vi "KEVIN CREATE EMAIL.vi"(9 "DATA IN":T2, 10 "BYU ID # IN":string, 11 "connection reference in":T3) -> (2 "MESSAGE OUT":string, 3 "connection reference out":T3)   [LabVIEW 2019]
uses:
  <vilib>/addons/database/Connection.llb/Conn ObjectReference.ctl
  Controls/Table Data Types/Inventory Data Type.ctl
  Controls/Table Data Types/User Data Type.ctl
  <vilib>/addons/database/_DB Variant To Data/Database Variant To Data.xnode
  <vilib>/addons/database/NI_Database_API.lvlib
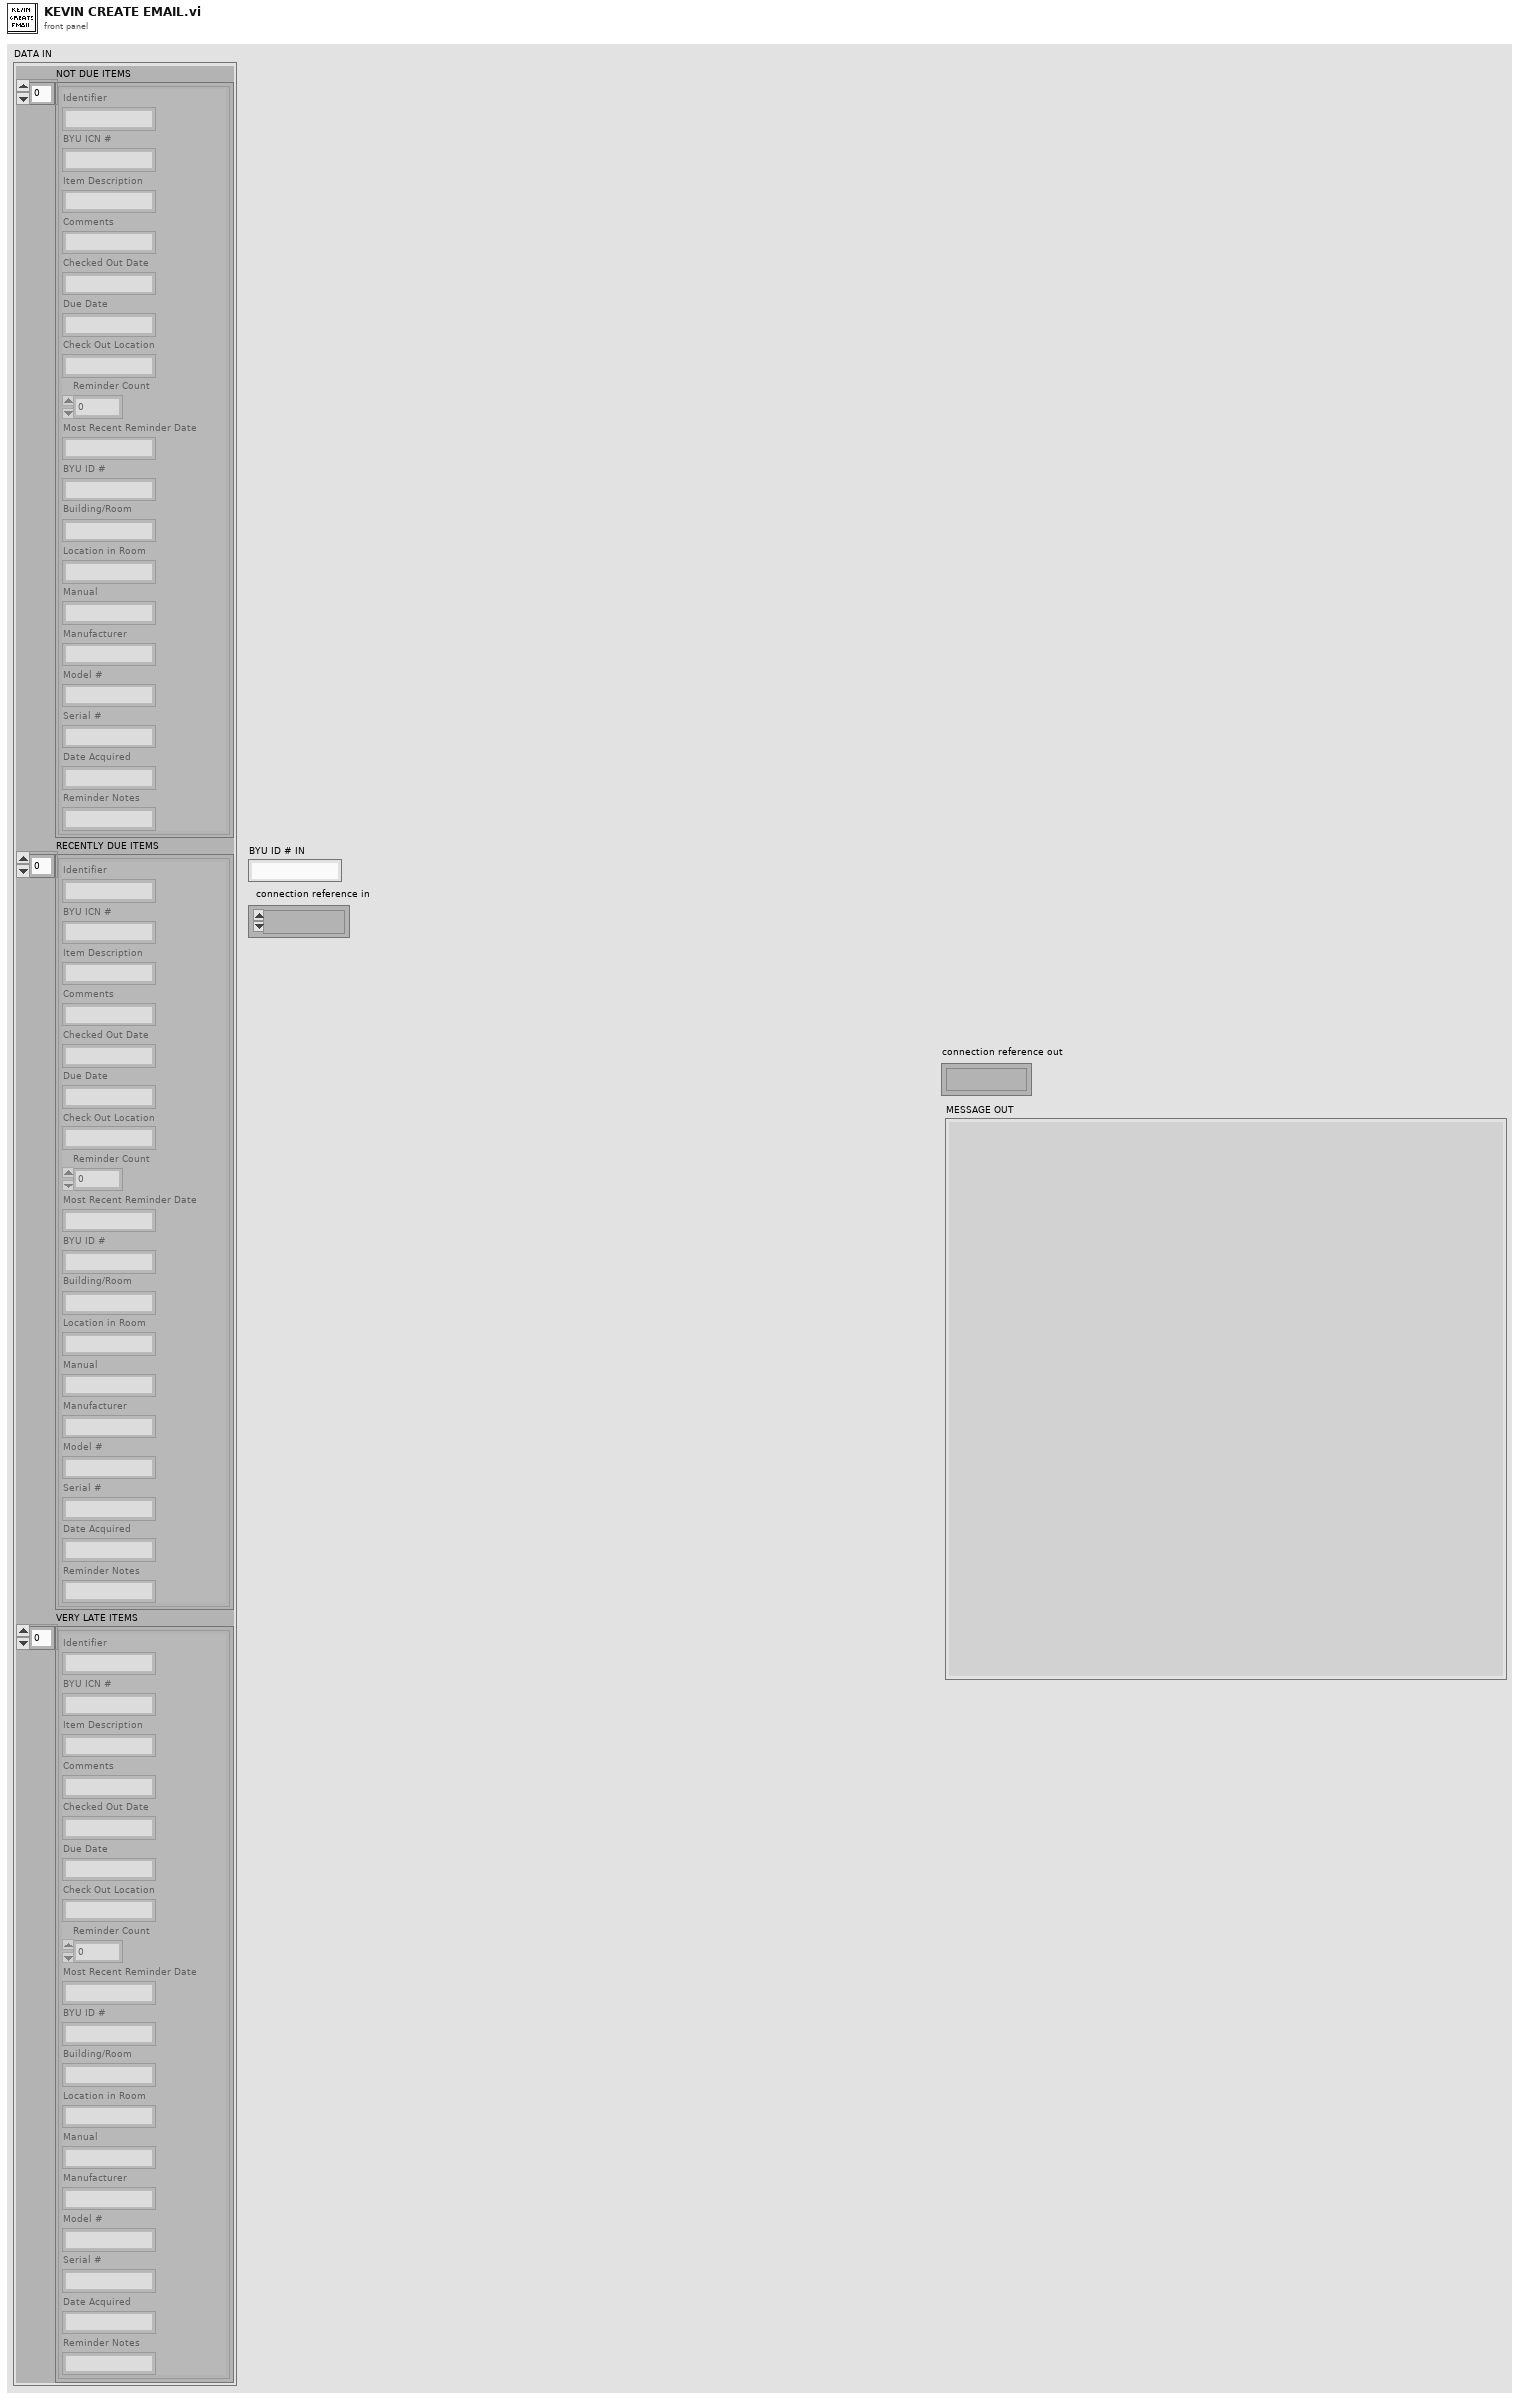
[diagram p1: front panel]
types:
  T1 = typedef "Inventory Data Type.ctl" = cluster{"Identifier":string, "BYU ICN #":string, "Item Description":string, "Comments":string, "Checked Out Date":string, "Due Date":string, "Check Out Location":string, "Reminder Count":i32, "Most Recent Reminder Date":string, "BYU ID #":string, "Building/Room":string, "Location in Room":string, "Manual":string, "Manufacturer":string, "Model #":string, "Serial #":string, "Date Acquired":string, "Reminder Notes":string}
  T2 = cluster{"NOT DUE ITEMS":T1[], "RECENTLY DUE ITEMS":T1[], "VERY LATE ITEMS":T1[]}
  T3 = typedef "NI_Database_API.lvlib/Conn ObjectReference.ctl" = refnum<k1>
  T4 = typedef "User Data Type.ctl" = cluster{"BYU ID #":string, "First Name":string, "Last Name":string, "Phone Number":string, "Email":string, "Department":string, "Graduation Status":string, "Anticipated Graduation Year":string, "Credit Score":dbl, "Date Added":string, "Graduation Clearance Date":string, "Picture File Name":string, "User Comments":string}
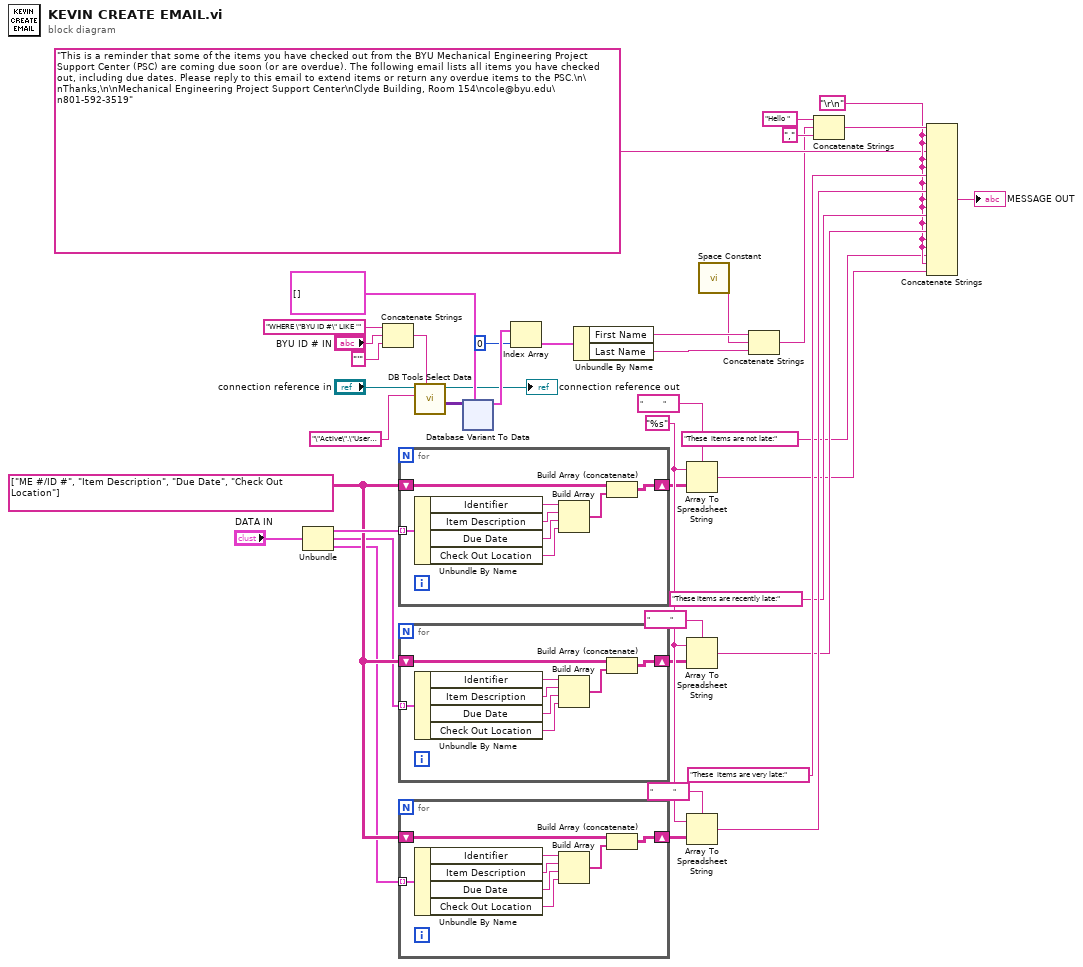
[diagram p0: block diagram]
diagram:
  w17 = "%s" ("table")
  w19 = "\r\n"
  w25 = string[][] [["ME #/ID #", "Item Description", "Due Date", "Check Out Location"]]
  n1 = Unbundle("DATA IN") -> ("NOT DUE ITEMS"=w26:T1[], "RECENTLY DUE ITEMS"=w3:T1[], "VERY LATE ITEMS"=w4:T1[])
  n2 = Concatenate Strings("WHERE \"BYU ID #\" LIKE '" ("table"), "BYU ID # IN", "'" ("table")) -> (w35:string)
  n3 = for {
    tunnel: w26 -> [w48] mode=indexing
    shift-right: [w41] -> w16
    shift-left: w25 -> [w43]
    n4 = Unbundle By Name(w48) -> ("Identifier"=w47:string, "Item Description"=w46:string, "Due Date"=w45:string, "Check Out Location"=w44:string)
    n5 = Build Array(w47, w46, w45, w44) -> (w42:string[])
    n6 = Build Array (concatenate)(w43, w42) -> (w41:string[][])
  }
  n7 = for {
    tunnel: w3 -> [w56] mode=indexing
    shift-right: [w49] -> w15
    shift-left: w25 -> [w51]
    n8 = Unbundle By Name(w56) -> ("Identifier"=w55:string, "Item Description"=w54:string, "Due Date"=w53:string, "Check Out Location"=w52:string)
    n9 = Build Array(w55, w54, w53, w52) -> (w50:string[])
    n10 = Build Array (concatenate)(w51, w50) -> (w49:string[][])
  }
  n11 = for {
    tunnel: w4 -> [w64] mode=indexing
    shift-right: [w57] -> w14
    shift-left: w25 -> [w59]
    n12 = Unbundle By Name(w64) -> ("Identifier"=w63:string, "Item Description"=w62:string, "Due Date"=w61:string, "Check Out Location"=w60:string)
    n13 = Build Array(w63, w62, w61, w60) -> (w58:string[])
    n14 = Build Array (concatenate)(w59, w58) -> (w57:string[][])
  }
  n15 = call <vilib>:"DB Tools Select Data.vi"("condition"=w35, "table"="\"Active\".\"Users\"", "connection reference"="connection reference in") -> ("data"=w34:variant[][], "connection reference out"=→"connection reference out":T3)  [unwired: 3 in, 1 out]
  n16 = xnode "Database Variant To Data"("database variant"=w34, "type"=T4[] [] ("Array")) -> ("data"=w32:T4[])  [unwired: 1 in, 1 out]
  n17 = Index Array(array=w32, index=0) -> (element=w30:T4)
  n18 = Unbundle By Name(w30) -> ("First Name"=w7:string, "Last Name"=w8:string)
  n19 = Array To Spreadsheet String(delimiter (Tab)="          ", array=w16, 3:w17) -> (spreadsheet string=w1:string)
  n20 = Array To Spreadsheet String(delimiter (Tab)="          ", array=w15, 3:w17) -> (spreadsheet string=w20:string)
  n21 = Array To Spreadsheet String(delimiter (Tab)="          ", array=w14, 3:w17) -> (spreadsheet string=w22:string)
  n22 = call <vilib>:"Space Constant.vi"() -> ("String"=w6:string)
  n23 = Concatenate Strings(w7, w6, w8) -> (w5:string)
  n24 = Concatenate Strings("Hello " ("table"), w5, "," ("table")) -> (w24:string)
  n25 = Concatenate Strings(w24, w19, w19, "This is a reminder that some of the items you have checked out from the BYU Mechanical Engineering Project Support Center (PSC) are coming due soon (or are overdue). The following email lists all items you have checked out, including due dates. Please reply to this email to extend items or return any overdue items to the PSC.\n\nThanks,\n\nMechanical Engineering Project Support Center\nClyde Building, Room 154\ncole@byu.edu\n801-592-3519" ("table"), w19, w19, "These  items are very late:" ("table"), w19, w22, w19, w19, "These items are recently late:" ("table"), w19, w20, w19, w19, "These  items are not late:" ("table"), w19, w1) -> (→"MESSAGE OUT":string)
